vi "2D Inverse FFT.vi"(1 "X":cdb[][](array[numeric]) format="%.2f") -> (0 "FFT {X}":dbl[][](array[numeric]) format="%.2f")   [LabVIEW 2024]
uses:
  <vilib>/Analysis/2dsp.llb/Inverse Complex FFT.vi
  <vilib>/Analysis/2dsp.llb/Inverse Real FFT.vi
  <vilib>/Analysis/NI_AALPro.lvlib
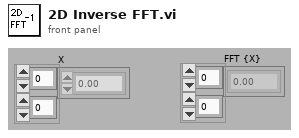
[diagram p1: front panel]
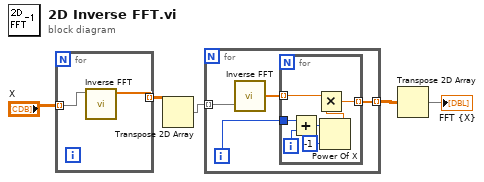
[diagram p0: block diagram]
diagram:
  n1 = for {
    tunnel: "X" -> [w7] mode=indexing
    tunnel: [w6] -> w3 mode=indexing
    n2 = call-poly <vilib>:"Inverse FFT.vi"("FFT {X}"=w7) -> ("X"=w6:cdb[])  [unwired: 9 in, 1 out]
  }
  n3 = Transpose 2D Array(2D array=w3) -> (transposed array=w4:cdb[][])
  n4 = for {
    tunnel: w4 -> [w11] mode=indexing
    tunnel: [w9] -> w5 mode=indexing
    i -> [w8]
    n5 = call-poly <vilib>:"Inverse FFT.vi"("FFT {X}"=w11) -> ("X"=w10:dbl[])  [unwired: 9 in, 1 out]
    n6 = for {
      tunnel: w8 -> [w17]
      tunnel: w10 -> [w13] mode=indexing
      tunnel: [w12] -> w9 mode=indexing
      i -> [w18]
      n7 = Add(x=w17, y=w18) -> (x+y=w16:i32)
      n8 = Power Of X(1:-1, 2:w16) -> (0:w14:dbl)
      n9 = Multiply(x=w13, y=w14) -> (x*y=w12:dbl)
    }
  }
  n10 = Transpose 2D Array(2D array=w5) -> (transposed array=→"FFT {X}":dbl[][])
